vi "Retrieve Eyes OC Montage.vi"(11 "ListBox in":refnum<vi>) -> (1 "Valid?":bool, 2 "Value":i32, 3 "EEG Channels":T1(array[cluster]))   [LabVIEW 2016, in "Settings Editor.lvlib"]
uses:
  Settings Editor.lvlib
  CML Shared/EEG Channel Settings.ctl
  <vilib>/Utility/xml.llb/Read From XML File(string).vi
  CML Shared/CML Shared.lvlib
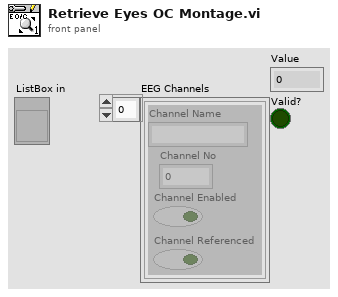
[diagram p1: front panel]
types:
  T1 = cluster{"Channel Name":string, "Channel No":u8, "Channel Enabled":bool, "Channel Referenced":bool}[]
  T2 = typedef "CML Shared.lvlib/EEG Channel Settings.ctl" = cluster{"16 EEG Channels":cluster{"Channel Name":string, "Channel No":u8, "Channel Enabled":bool, "Channel Referenced":bool}[], "Gain":u8}
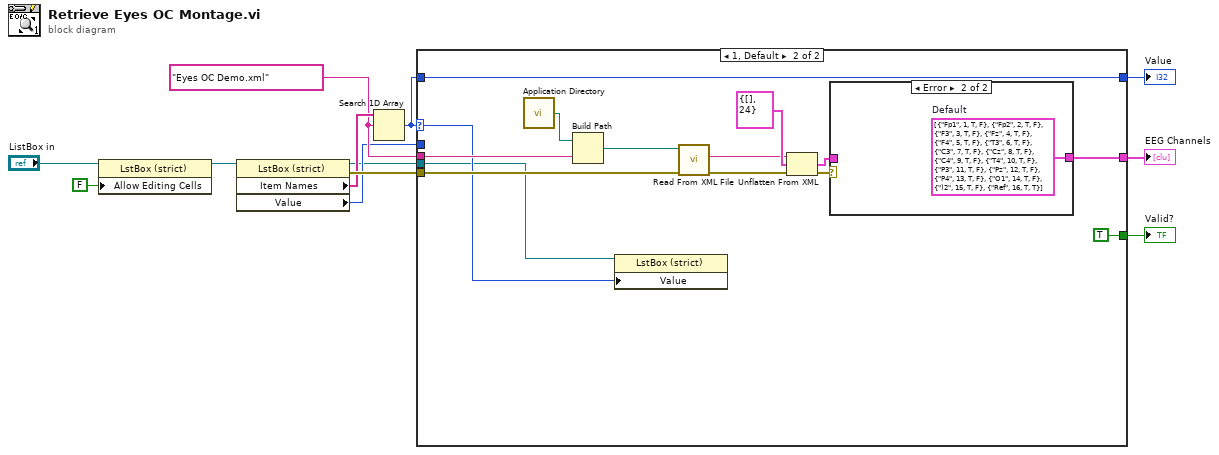
[diagram p0: block diagram]
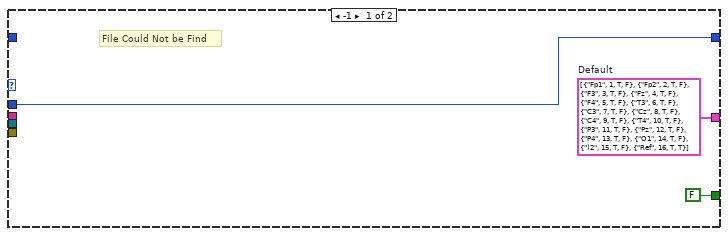
[diagram p2: hidden frame]
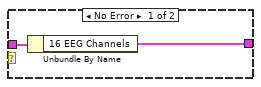
[diagram p3: hidden frame]
diagram:
  w6 = "Eyes OC Demo.xml"
  n1 = property class="LstBox (strict)"(reference="ListBox in", "Allow Editing Cells"=FALSE) -> (reference out=w10:refnum<vi>)  [unwired: 1 in, 1 out]
  n2 = property class="LstBox (strict)"(reference=w10) -> (reference out=w1:refnum<vi>, error out=w11:errorcluster, "Item Names"=w7:string[], "Value"=w3:i32)  [unwired: 1 in]
  n3 = Search 1D Array(1D array=w7, element=w6) -> (index of element=w5:i32)  [unwired: 1 in]
  n4 = case shown="1, Default" w5 {
    selector: w5 -> [_ w17]
    tunnel: [w14 w28] -> w12
    tunnel: w11 -> [_ w25]
    tunnel: w6 -> [_ w20]
    tunnel: w5 -> [_ w19]
    tunnel: [w15 w19] -> w4
    tunnel: w3 -> [w15 _]
    tunnel: [FALSE TRUE] -> w2
    tunnel: w1 -> [_ w16]
    frame -1 {
      w14 = T1 [{"Channel Name"="Fp1", "Channel No"=1, "Channel Enabled"=TRUE, "Channel Referenced"=FALSE}, {"Channel Name"="Fp2", "Channel No"=2, "Channel Enabled"=TRUE, "Channel Referenced"=FALSE}, {"Channel Name"="F3", "Channel No"=3, "Channel Enabled"=TRUE, "Channel Referenced"=FALSE}, {"Channel Name"="Fz", "Channel No"=4, "Channel Enabled"=TRUE, "Channel Referenced"=FALSE}, {"Channel Name"="F4", "Channel No"=5, "Channel Enabled"=TRUE, "Channel Referenced"=FALSE}, {"Channel Name"="T3", "Channel No"=6, "Channel Enabled"=TRUE, "Channel Referenced"=FALSE}, {"Channel Name"="C3", "Channel No"=7, "Channel Enabled"=TRUE, "Channel Referenced"=FALSE}, {"Channel Name"="Cz", "Channel No"=8, "Channel Enabled"=TRUE, "Channel Referenced"=FALSE}, {"Channel Name"="C4", "Channel No"=9, "Channel Enabled"=TRUE, "Channel Referenced"=FALSE}, {"Channel Name"="T4", "Channel No"=10, "Channel Enabled"=TRUE, "Channel Referenced"=FALSE}, {"Channel Name"="P3", "Channel No"=11, "Channel Enabled"=TRUE, "Channel Referenced"=FALSE}, {"Channel Name"="Pz", "Channel No"=12, "Channel Enabled"=TRUE, "Channel Referenced"=FALSE}, {"Channel Name"="P4", "Channel No"=13, "Channel Enabled"=TRUE, "Channel Referenced"=FALSE}, {"Channel Name"="O1", "Channel No"=14, "Channel Enabled"=TRUE, "Channel Referenced"=FALSE}, {"Channel Name"=")2", "Channel No"=15, "Channel Enabled"=TRUE, "Channel Referenced"=FALSE}, {"Channel Name"="Ref", "Channel No"=16, "Channel Enabled"=TRUE, "Channel Referenced"=TRUE}]  # Default
      # "File Could Not be Find"
    }
    frame 1, Default {
      n5 = call <vilib>:"Application Directory.vi"() -> ("Application Directory"=w21:path)
      n6 = Build Path(base path=w21, name or relative path=w20) -> (appended path=w24:path)
      n7 = property class="LstBox (strict)"(reference=w16, "Value"=w17) -> ()  [unwired: 1 in, 2 out]
      n8 = call-poly <vilib>:"Read From XML File.vi"("error in (no error)"=w25, "XML File Path"=w24) -> ("error out"=w23:errorcluster, "XML Elements"=w22:string)  [unwired: 7 in, 1 out]
      n9 = Unflatten From XML(xml string=w22, type=T2 {"16 EEG Channels"=[], "Gain"=24} ("EEG Channels"), error in (no error)=w23) -> (value=w27:T2, error out=w29:errorcluster)
      n10 = case shown="Error" w29 {
        tunnel: w27 -> [w31 _]
        tunnel: [w30 w32] -> w28
        frame No Error {
          n11 = Unbundle By Name(w31) -> ("16 EEG Channels"=w30:T1)
        }
        frame Error {
          w32 = T1 [{"Channel Name"="Fp1", "Channel No"=1, "Channel Enabled"=TRUE, "Channel Referenced"=FALSE}, {"Channel Name"="Fp2", "Channel No"=2, "Channel Enabled"=TRUE, "Channel Referenced"=FALSE}, {"Channel Name"="F3", "Channel No"=3, "Channel Enabled"=TRUE, "Channel Referenced"=FALSE}, {"Channel Name"="Fz", "Channel No"=4, "Channel Enabled"=TRUE, "Channel Referenced"=FALSE}, {"Channel Name"="F4", "Channel No"=5, "Channel Enabled"=TRUE, "Channel Referenced"=FALSE}, {"Channel Name"="T3", "Channel No"=6, "Channel Enabled"=TRUE, "Channel Referenced"=FALSE}, {"Channel Name"="C3", "Channel No"=7, "Channel Enabled"=TRUE, "Channel Referenced"=FALSE}, {"Channel Name"="Cz", "Channel No"=8, "Channel Enabled"=TRUE, "Channel Referenced"=FALSE}, {"Channel Name"="C4", "Channel No"=9, "Channel Enabled"=TRUE, "Channel Referenced"=FALSE}, {"Channel Name"="T4", "Channel No"=10, "Channel Enabled"=TRUE, "Channel Referenced"=FALSE}, {"Channel Name"="P3", "Channel No"=11, "Channel Enabled"=TRUE, "Channel Referenced"=FALSE}, {"Channel Name"="Pz", "Channel No"=12, "Channel Enabled"=TRUE, "Channel Referenced"=FALSE}, {"Channel Name"="P4", "Channel No"=13, "Channel Enabled"=TRUE, "Channel Referenced"=FALSE}, {"Channel Name"="O1", "Channel No"=14, "Channel Enabled"=TRUE, "Channel Referenced"=FALSE}, {"Channel Name"=")2", "Channel No"=15, "Channel Enabled"=TRUE, "Channel Referenced"=FALSE}, {"Channel Name"="Ref", "Channel No"=16, "Channel Enabled"=TRUE, "Channel Referenced"=TRUE}]  # Default
        }
      }
    }
  }
  "EEG Channels" <- w12
  "Value" <- w4
  "Valid?" <- w2
